vi "Parse OSF Project.vi"(8 "error in":errorcluster, 11 "Project JSON":string="{\"data\":{\"id\":\"xecwn\",\"type\":\"nodes\",\"attributes\":{\"title\":\"Pressure-driven quantum magneto-transport phenomena in topological semimetals\",\"description\":\"\",\"category\":\"\",\"custom_citation\":null,\"date_created\":\"2020-12-07T03:50:06.257212\",\"date_modified\":\"2020-12-07T03:50:06.257212\",\"registration\":false,\"preprint\":false,\"fork\":false,\"collection\":false,\"tags\":[],\"access_requests_enabled\":true,\"node_license\":null,\"current_user_can_comment\":true,\"current_user_permissions\":[\"admin\",\"write\",\"read\"],\"current_user_is_contributor\":true,\"current_user_is_contributor_or_group_member\":true,\"wiki_enabled\":true,\"public\":false,\"subjects\":[]},\"relationships\":{\"children\":{\"links\":{\"related\":{\"href\":\"https://api.osf.io/v2/nodes/xecwn/children/\",\"meta\":{}}}},\"comments\":{\"links\":{\"related\":{\"href\":\"https://api.osf.io/v2/nodes/xecwn/comments/?filter%5Btarget%5D=xecwn\",\"meta\":{}}}},\"contributors\":{\"links\":{\"related\":{\"href\":\"https://api.osf.io/v2/nodes/xecwn/contributors/\",\"meta\":{}}}},\"bibliographic_contributors\":{\"links\":{\"related\":{\"href\":\"https://api.osf.io/v2/nodes/xecwn/bibliographic_contributors/\",\"meta\":{}}}},\"implicit_contributors\":{\"links\":{\"related\":{\"href\":\"https://api.osf.io/v2/nodes/xecwn/implicit_contributors/\",\"meta\":{}}}},\"files\":{\"links\":{\"related\":{\"href\":\"https://api.osf.io/v2/nodes/xecwn/files/\",\"meta\":{}}}},\"settings\":{\"links\":{\"related\":{\"href\":\"https://api.osf.io/v2/nodes/xecwn/settings/\",\"meta\":{}}},\"data\":{\"id\":\"xecwn\",\"type\":\"nodes\"}},\"wikis\":{\"links\":{\"related\":{\"href\":\"https://api.osf.io/v2/nodes/xecwn/wikis/\",\"meta\":{}}}},\"forks\":{\"links\":{\"related\":{\"href\":\"https://api.osf.io/v2/nodes/xecwn/forks/\",\"meta\":{}}}},\"groups\":{\"links\":{\"related\":{\"href\":\"https://api.osf.io/v2/nodes/xecwn/groups/\",\"meta\":{}}}},\"node_links\":{\"links\":{\"related\":{\"href\":\"https://api.osf.io/v2/nodes/xecwn/node_links/\",\"meta\":{}}}},\"linked_by_nodes\":{\"links\":{\"related\":{\"href\":\"https://api.osf.io/v2/nodes/xecwn/linked_by_nodes/\",\"meta\":{}}}},\"linked_by_registrations\":{\"links\":{\"related\":{\"href\":\"https://api.osf.io/v2/nodes/xecwn/linked_by_registrations/\",\"meta\":{}}}},\"identifiers\":{\"links\":{\"related\":{\"href\":\"https://api.osf.io/v2/nodes/xecwn/identifiers/\",\"meta\":{}}}},\"affiliated_institutions\":{\"links\":{\"related\":{\"href\":\"https://api.osf.io/v2/nodes/xecwn/institutions/\",\"meta\":{}},\"self\":{\"href\":\"https://api.osf.io/v2/nodes/xecwn/relationships/institutions/\",\"meta\":{}}}},\"draft_registrations\":{\"links\":{\"related\":{\"href\":\"https://api.osf.io/v2/nodes/xecwn/draft_registrations/\",\"meta\":{}}}},\"registrations\":{\"links\":{\"related\":{\"href\":\"https://api.osf.io/v2/nodes/xecwn/registrations/\",\"meta\":{}}}},\"region\":{\"links\":{\"related\":{\"href\":\"https://api.osf.io/v2/regions/us/\",\"meta\":{}}},\"data\":{\"id\":\"us\",\"type\":\"regions\"}},\"root\":{\"links\":{\"related\":{\"href\":\"https://api.osf.io/v2/nodes/xecwn/\",\"meta\":{}}},\"data\":{\"id\":\"xecwn\",\"type\":\"nodes\"}},\"logs\":{\"links\":{\"related\":{\"href\":\"https://api.osf.io/v2/nodes/xecwn/logs/\",\"meta\":{}}}},\"linked_nodes\":{\"links\":{\"related\":{\"href\":\"https://api.osf.io/v2/nodes/xecwn/linked_nodes/\",\"meta\":{}},\"self\":{\"href\":\"https://api.osf.io/v2/nodes/xecwn/relationships/linked_nodes/\",\"meta\":{}}}},\"linked_registrations\":{\"links\":{\"related\":{\"href\":\"https://api.osf.io/v2/nodes/xecwn/linked_registrations/\",\"meta\":{}},\"self\":{\"href\":\"https://api.osf.io/v2/nodes/xecwn/relationships/linked_registrations/\",\"meta\":{}}}},\"view_only_links\":{\"links\":{\"related\":{\"href\":\"https://api.osf.io/v2/nodes/xecwn/view_only_links/\",\"meta\":{}}}},\"citation\":{\"links\":{\"related\":{\"href\":\"https://api.osf.io/v2/nodes/xecwn/citation/\",\"meta\":{}}},\"data\":{\"id\":\"xecwn\",\"type\":\"nodes\"}},\"preprints\":{\"links\":{\"related\":{\"href\":\"https://api.osf.io/v2/nodes/xecwn/preprints/\",\"meta\":{}}}},\"storage\":{\"links\":{\"related\":{\"href\":\"https://api.osf.io/v2/nodes/xecwn/storage/\",\"meta\":{}}},\"data\":{\"id\":\"xecwn\",\"type\":\"nodes\"}}},\"links\":{\"html\":\"https://osf.io/xecwn/\",\"self\":\"https://api.osf.io/v2/nodes/xecwn/\"}},\"meta\":{\"version\":\"2.0\"}}") -> (0 "error out":errorcluster, 2 "Wiki href":string, 3 "Project ID":string)   [LabVIEW 2020]
uses:
  <vilib>/JDP Science/JSONtext/JSONtext.lvlib
panel:
  out "Found":bool
  out "Formated JSON":string="{\"data\":{\"id\":\"xecwn\",\"type\":\"nodes\",\"attributes\":{\"title\":\"Pressure-driven quantum magneto-transport phenomena in topological semimetals\",\"description\":\"\",\"category\":\"\",\"custom_citation\":null,\"date_created\":\"2020-12-07T03:50:06.257212\",\"date_modified\":\"2020-12-07T03:50:06.257212\",\"registration\":false,\"preprint\":false,\"fork\":false,\"collection\":false,\"tags\":[],\"access_requests_enabled\":true,\"node_license\":null,\"current_user_can_comment\":true,\"current_user_permissions\":[\"admin\",\"write\",\"read\"],\"current_user_is_contributor\":true,\"current_user_is_contributor_or_group_member\":true,\"wiki_enabled\":true,\"public\":false,\"subjects\":[]},\"relationships\":{\"children\":{\"links\":{\"related\":{\"href\":\"https://api.osf.io/v2/nodes/xecwn/children/\",\"meta\":{}}}},\"comments\":{\"links\":{\"related\":{\"href\":\"https://api.osf.io/v2/nodes/xecwn/comments/?filter%5Btarget%5D=xecwn\",\"meta\":{}}}},\"contributors\":{\"links\":{\"related\":{\"href\":\"https://api.osf.io/v2/nodes/xecwn/contributors/\",\"meta\":{}}}},\"bibliographic_contributors\":{\"links\":{\"related\":{\"href\":\"https://api.osf.io/v2/nodes/xecwn/bibliographic_contributors/\",\"meta\":{}}}},\"implicit_contributors\":{\"links\":{\"related\":{\"href\":\"https://api.osf.io/v2/nodes/xecwn/implicit_contributors/\",\"meta\":{}}}},\"files\":{\"links\":{\"related\":{\"href\":\"https://api.osf.io/v2/nodes/xecwn/files/\",\"meta\":{}}}},\"settings\":{\"links\":{\"related\":{\"href\":\"https://api.osf.io/v2/nodes/xecwn/settings/\",\"meta\":{}}},\"data\":{\"id\":\"xecwn\",\"type\":\"nodes\"}},\"wikis\":{\"links\":{\"related\":{\"href\":\"https://api.osf.io/v2/nodes/xecwn/wikis/\",\"meta\":{}}}},\"forks\":{\"links\":{\"related\":{\"href\":\"https://api.osf.io/v2/nodes/xecwn/forks/\",\"meta\":{}}}},\"groups\":{\"links\":{\"related\":{\"href\":\"https://api.osf.io/v2/nodes/xecwn/groups/\",\"meta\":{}}}},\"node_links\":{\"links\":{\"related\":{\"href\":\"https://api.osf.io/v2/nodes/xecwn/node_links/\",\"meta\":{}}}},\"linked_by_nodes\":{\"links\":{\"related\":{\"href\":\"https://api.osf.io/v2/nodes/xecwn/linked_by_nodes/\",\"meta\":{}}}},\"linked_by_registrations\":{\"links\":{\"related\":{\"href\":\"https://api.osf.io/v2/nodes/xecwn/linked_by_registrations/\",\"meta\":{}}}},\"identifiers\":{\"links\":{\"related\":{\"href\":\"https://api.osf.io/v2/nodes/xecwn/identifiers/\",\"meta\":{}}}},\"affiliated_institutions\":{\"links\":{\"related\":{\"href\":\"https://api.osf.io/v2/nodes/xecwn/institutions/\",\"meta\":{}},\"self\":{\"href\":\"https://api.osf.io/v2/nodes/xecwn/relationships/institutions/\",\"meta\":{}}}},\"draft_registrations\":{\"links\":{\"related\":{\"href\":\"https://api.osf.io/v2/nodes/xecwn/draft_registrations/\",\"meta\":{}}}},\"registrations\":{\"links\":{\"related\":{\"href\":\"https://api.osf.io/v2/nodes/xecwn/registrations/\",\"meta\":{}}}},\"region\":{\"links\":{\"related\":{\"href\":\"https://api.osf.io/v2/regions/us/\",\"meta\":{}}},\"data\":{\"id\":\"us\",\"type\":\"regions\"}},\"root\":{\"links\":{\"related\":{\"href\":\"https://api.osf.io/v2/nodes/xecwn/\",\"meta\":{}}},\"data\":{\"id\":\"xecwn\",\"type\":\"nodes\"}},\"logs\":{\"links\":{\"related\":{\"href\":\"https://api.osf.io/v2/nodes/xecwn/logs/\",\"meta\":{}}}},\"linked_nodes\":{\"links\":{\"related\":{\"href\":\"https://api.osf.io/v2/nodes/xecwn/linked_nodes/\",\"meta\":{}},\"self\":{\"href\":\"https://api.osf.io/v2/nodes/xecwn/relationships/linked_nodes/\",\"meta\":{}}}},\"linked_registrations\":{\"links\":{\"related\":{\"href\":\"https://api.osf.io/v2/nodes/xecwn/linked_registrations/\",\"meta\":{}},\"self\":{\"href\":\"https://api.osf.io/v2/nodes/xecwn/relationships/linked_registrations/\",\"meta\":{}}}},\"view_only_links\":{\"links\":{\"related\":{\"href\":\"https://api.osf.io/v2/nodes/xecwn/view_only_links/\",\"meta\":{}}}},\"citation\":{\"links\":{\"related\":{\"href\":\"https://api.osf.io/v2/nodes/xecwn/citation/\",\"meta\":{}}},\"data\":{\"id\":\"xecwn\",\"type\":\"nodes\"}},\"preprints\":{\"links\":{\"related\":{\"href\":\"https://api.osf.io/v2/nodes/xecwn/preprints/\",\"meta\":{}}}},\"storage\":{\"links\":{\"related\":{\"href\":\"https://api.osf.io/v2/nodes/xecwn/storage/\",\"meta\":{}}},\"data\":{\"id\":\"xecwn\",\"type\":\"nodes\"}}},\"links\":{\"html\":\"https://osf.io/xecwn/\",\"self\":\"https://api.osf.io/v2/nodes/xecwn/\"}},\"meta\":{\"version\":\"2.0\"}}"
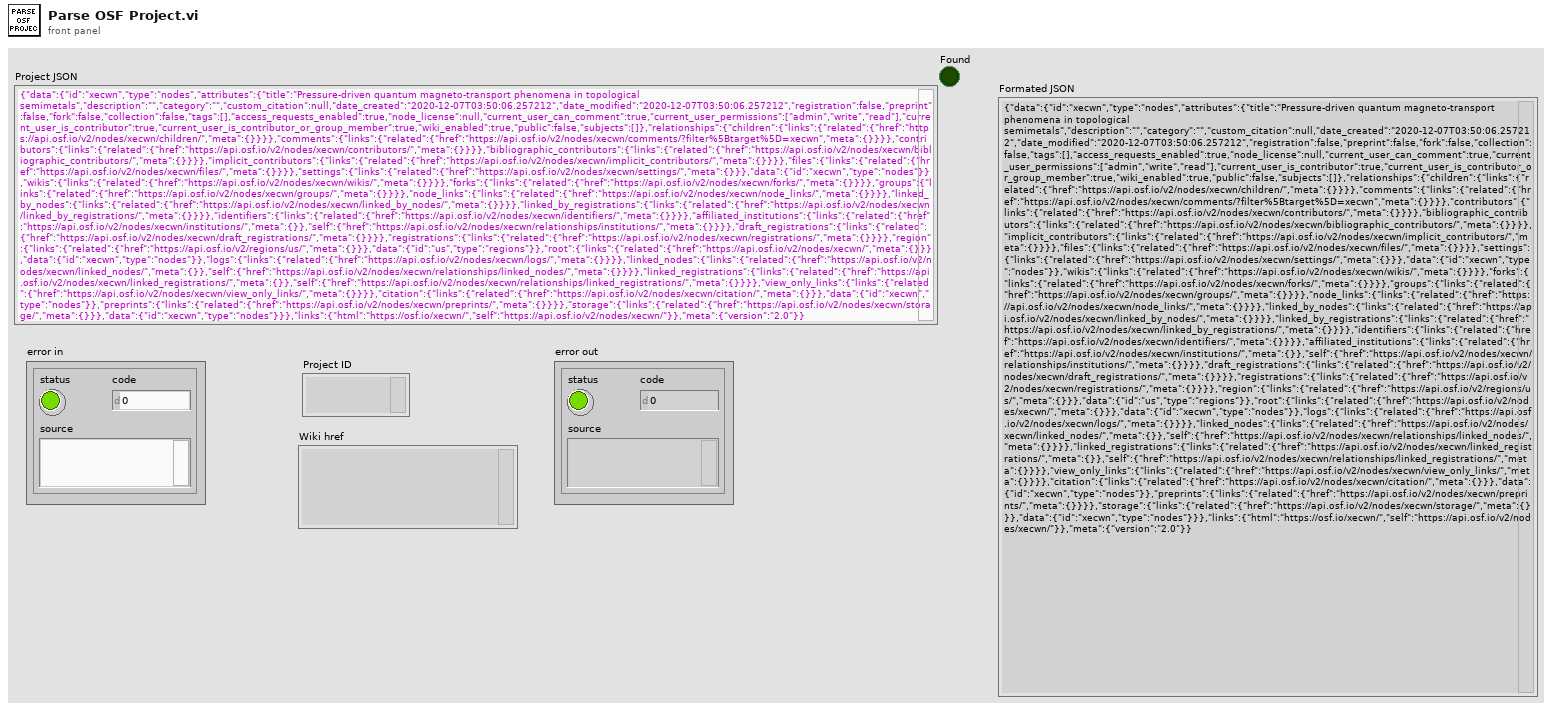
[diagram p1: front panel]
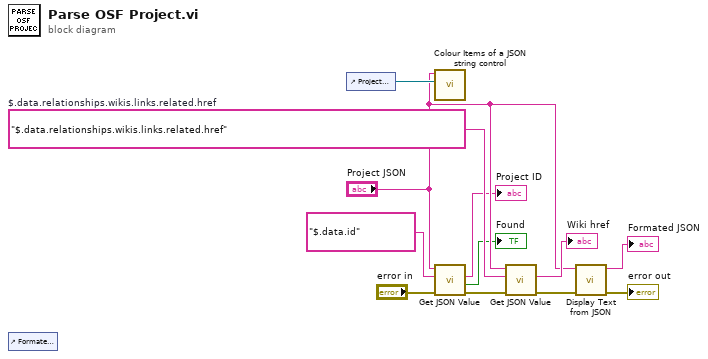
[diagram p0: block diagram]
diagram:
  w4 = "$.data.relationships.wikis.links.related.href"  # $.data.relationships.wikis.links.related.href
  n1 = control-ref of="Formated JSON"() -> ()  [unwired: 1 out]
  n2 = control-ref of="Project JSON"() -> (w11:refnum<vi>)
  n3 = call <vilib>:"Colour Items of a JSON string control.vi"("String Control"=w11, "JSON"="Project JSON") -> ()  [unwired: 10 in]
  n4 = call "Get JSON Value.vi"("error in"="error in", "$Path or Item Name"="$.data.id", "JSON in"="Project JSON") -> ("error out"=w8:errorcluster, "Found"=→"Found":bool, "String out"=→"Project ID":string)  [unwired: 4 in, 2 out]
  n5 = call "Get JSON Value.vi"("error in"=w8, "$Path or Item Name"=w4, "JSON in"="Project JSON") -> ("error out"=w7:errorcluster, "String out"=→"Wiki href":string)  [unwired: 4 in, 3 out]
  n6 = call <vilib>:"Display Text from JSON.vi"("error in (no error)"=w7, "Input JSON"="Project JSON") -> ("error out"=→"error out":errorcluster, "Display Text"=→"Formated JSON":string)  [unwired: 7 in, 1 out]
